vi "OPCClient.vi"() -> ()   [LabVIEW 2013]
doc: "This VI uses the DataSocket functions to read values from an OPC server. You can specify which URL you want to read. The National Instruments.OPCDemo server provides the possible OPC URLs for this example."
panel:
  in  "Go":bool
  out "Selected PR2 URL":string
  in  "Stop 2":bool
  in  "Next Position":i32[](array[numeric])
  out "Current Position":i32[](array[numeric])
  out "Selected CurPos URL":string
  in  "Stop":bool
  # "Overview: Demonstrates the use of the DataSocket functions to read data from an OPC server.\nRequirements: Windows\nInstructions:\n1. Run the VI.\n2. In the dialog that appears, select one of the demo OPC URLs under the Computer > National Instruments.OPCDemo > NI OPC Demo Server > Function Items category and click OK.\n3. The OPC Data chart will begin updating with values from the specified OPC URL.\n4. Click Stop to stop the VI."
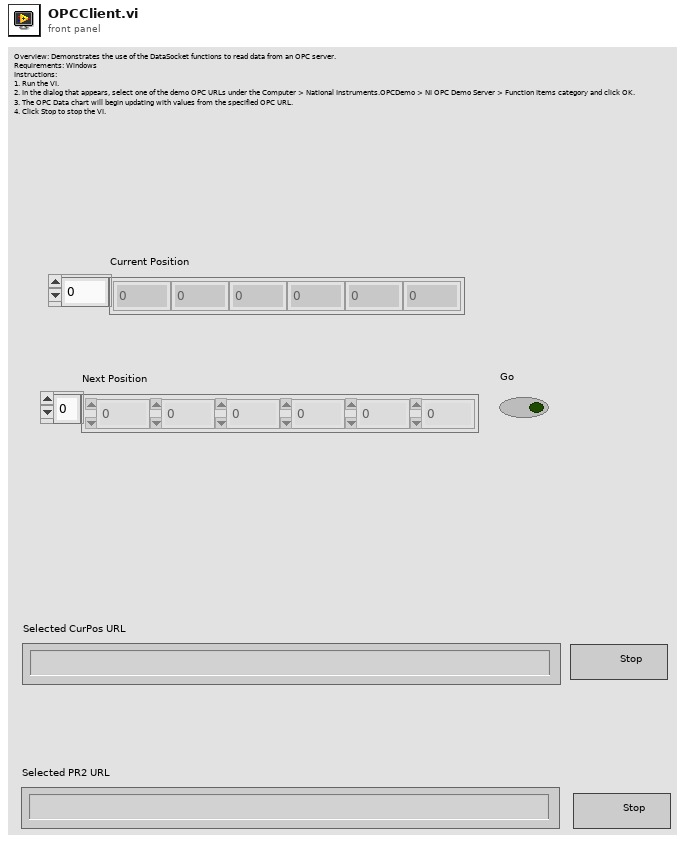
[diagram p1: front panel]
types:
  T1 = enum16{"Read", "Write", "ReadWrite", "BufferedRead", "BufferedReadWrite"}
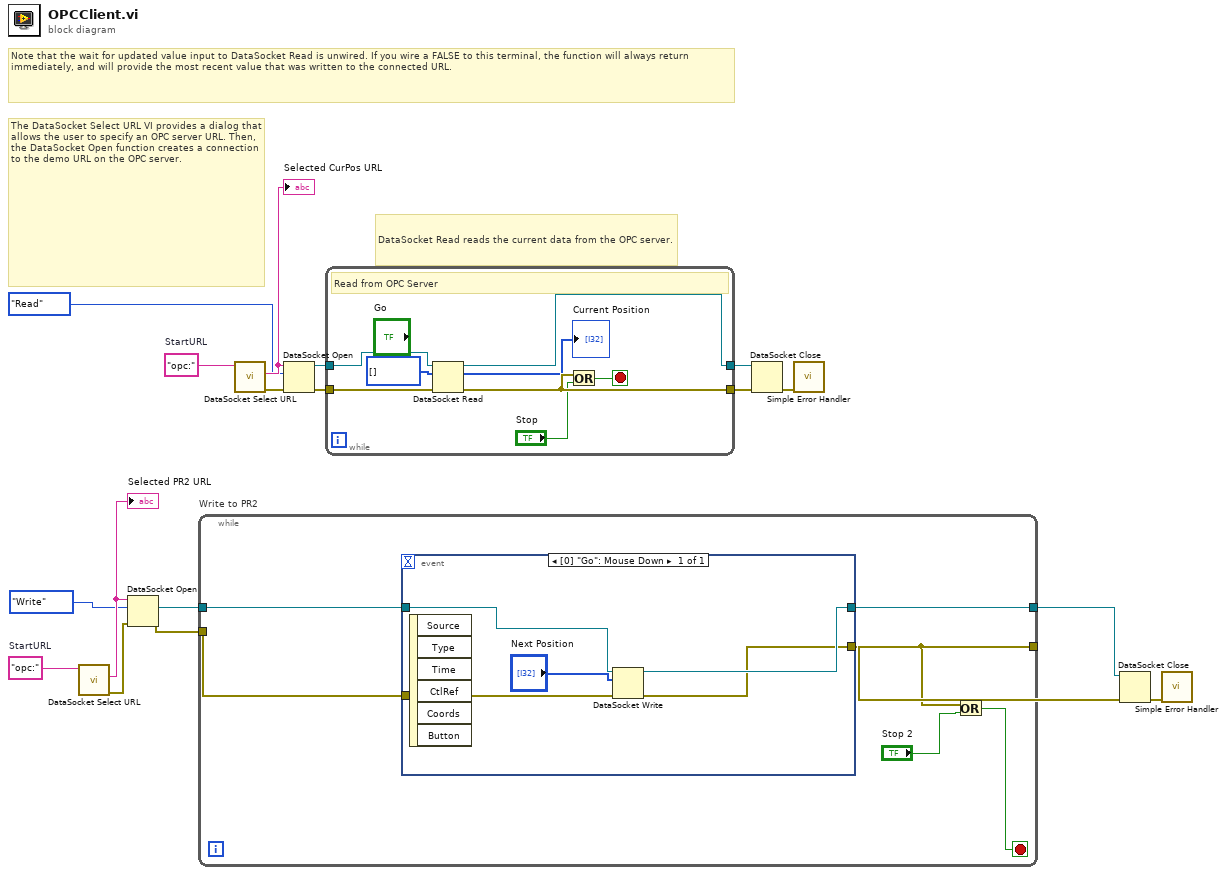
[diagram p0: block diagram]
diagram:
  w5 = "opc:"  # StartURL
  w11 = "opc:"  # StartURL
  # "Note that the wait for updated value input to DataSocket Read is unwired. If you wire a FALSE to this terminal, the function will always return immediately, and will provide the most recent value that was written to the connected URL."
  # "The DataSocket Select URL VI provides a dialog that allows the user to specify an OPC server URL. Then, the DataSocket Open function creates a connection to the demo URL on the OPC server."
  # "DataSocket Read reads the current data from the OPC server."
  n1 = call <vilib>:"DataSocket Select URL.vi"("StartURL (empty)"=w5) -> ("error out"=w4:errorcluster, "URL"=w3:string)  [unwired: 2 in, 7 out]
  "Selected PR2 URL" <- w3
  n2 = DataSocket Open(8:w4, 10:T1."Write" ("mode"), 11:w3) -> (0:w8:errorcluster, 3:w10:refnum<k13>)  [unwired: 1 out]
  n3 = while "Write to PR2" {
    tunnel: w10 -> [w24]
    tunnel: [w23] -> w9
    tunnel: w8 -> [w22]
    tunnel: [w20] -> w7
    stop <- w19 stop-if-true
    n4 = event shown="[0] \"Go\": Mouse Down" {
      selector: _ -> [_]
      dyn-events: _ -> [_]
      timeout: _ -> [_]
      tunnel: w24 -> [w29]
      tunnel: [w28] -> w23
      tunnel: w22 -> [w27]
      tunnel: [w26] -> w20
      event "Go": Mouse Down {
        n5 = event-data() -> ()  [unwired: 1 in, 6 out]
        n6 = DataSocket Write(8:w27, 10:"Next Position", 11:w29) -> (0:w26:errorcluster, 3:w28:refnum<k13>)  [unwired: 1 in, 1 out]
      }
    }
    n7 = Or(x=w20, y="Stop 2") -> (x .or. y?=w19:bool)
  }
  n8 = call <vilib>:"DataSocket Select URL.vi"("StartURL (empty)"=w11) -> ("error out"=w13:errorcluster, "URL"=w12:string)  [unwired: 2 in, 7 out]
  "Selected CurPos URL" <- w12
  n9 = DataSocket Open(8:w13, 10:T1."Read" ("mode"), 11:w12) -> (0:w16:errorcluster, 3:w18:refnum<k13>)  [unwired: 1 out]
  n10 = while {
    tunnel: [w33] -> w15
    tunnel: w16 -> [w35]
    tunnel: [w36] -> w17
    tunnel: w18 -> [w37]
    stop <- w34 stop-if-true
    # "Read from OPC Server"
    n11 = DataSocket Read(8:w35, 10:i32[] [] ("Array 2"), 11:w37) -> (0:w33:errorcluster, 2:→"Current Position":i32[], 3:w36:refnum<k13>)  [unwired: 6 out]
    n12 = Or(x=w33, y="Stop") -> (x .or. y?=w34:bool)
  }
  n13 = DataSocket Close(8:w15, 11:w17) -> (0:w14:errorcluster)  [unwired: 2 out]
  n14 = call <vilib>:"Simple Error Handler.vi"("error in (no error)"=w14) -> ()  [unwired: 4 in, 5 out]
  n15 = DataSocket Close(8:w7, 11:w9) -> (0:w6:errorcluster)  [unwired: 2 out]
  n16 = call <vilib>:"Simple Error Handler.vi"("error in (no error)"=w6) -> ()  [unwired: 4 in, 5 out]
